vi "init_main_panel.vi"(6 "Reset":refnum<vi>, 9 "Pause Button":refnum<vi>, 10 "Stop Button":refnum<vi>, 11 "Run":refnum<vi>) -> ()   [LabVIEW 2019]
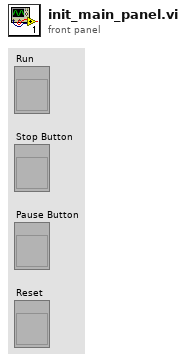
[diagram p1: front panel]
types:
  T1 = enum8{"Enabled", "Disabled", "Disabled and Grayed Out"}
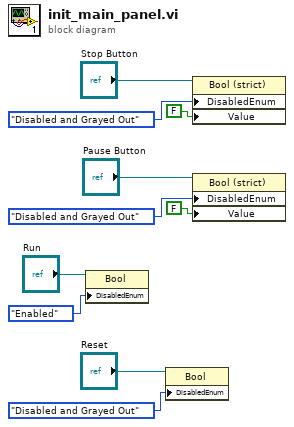
[diagram p0: block diagram]
diagram:
  n1 = property on="Property Node" class="Bool"(reference="Run", "DisabledEnum"=T1."Enabled" ("Disabled")) -> ()  [unwired: 1 in, 2 out]
  n2 = property on="Property Node" class="Bool"(reference="Reset", "DisabledEnum"=T1."Disabled and Grayed Out" ("Disabled")) -> ()  [unwired: 1 in, 2 out]
  n3 = property on="Property Node" class="Bool (strict)"(reference="Stop Button", "DisabledEnum"=T1."Disabled and Grayed Out" ("Disabled"), "Value"=FALSE ("Stop Button")) -> ()  [unwired: 1 in, 2 out]
  n4 = property on="Property Node" class="Bool (strict)"(reference="Pause Button", "DisabledEnum"=T1."Disabled and Grayed Out" ("Disabled"), "Value"=FALSE ("Pause Button")) -> ()  [unwired: 1 in, 2 out]
